vi "Mov_Avg_JS_Dual.vi"(6 "Cycle Length":dbl, 8 "Array In 2":dbl[](array[numeric]), 9 "Input 2":dbl, 10 "Array In":dbl[](array[numeric]), 11 "Input":dbl) -> (0 "Array Out Main 2":dbl[](array[numeric]), 1 "Mean 2":dbl format="%0.2f", 2 "Array Out Main":dbl[](array[numeric]), 3 "Mean":dbl format="%0.2f")   [LabVIEW 2014]
uses:
  <vilib>/Analysis/baseanly.llb/Mean (DBL).vi
  <vilib>/Analysis/NI_AALBase.lvlib
panel:
  # "Moving Average VI"
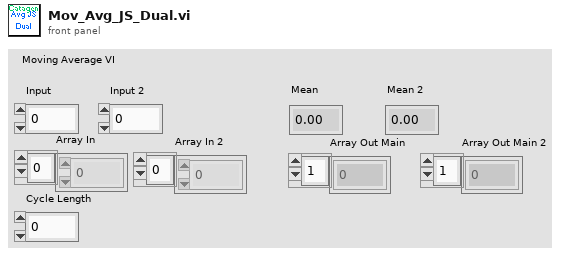
[diagram p1: front panel]
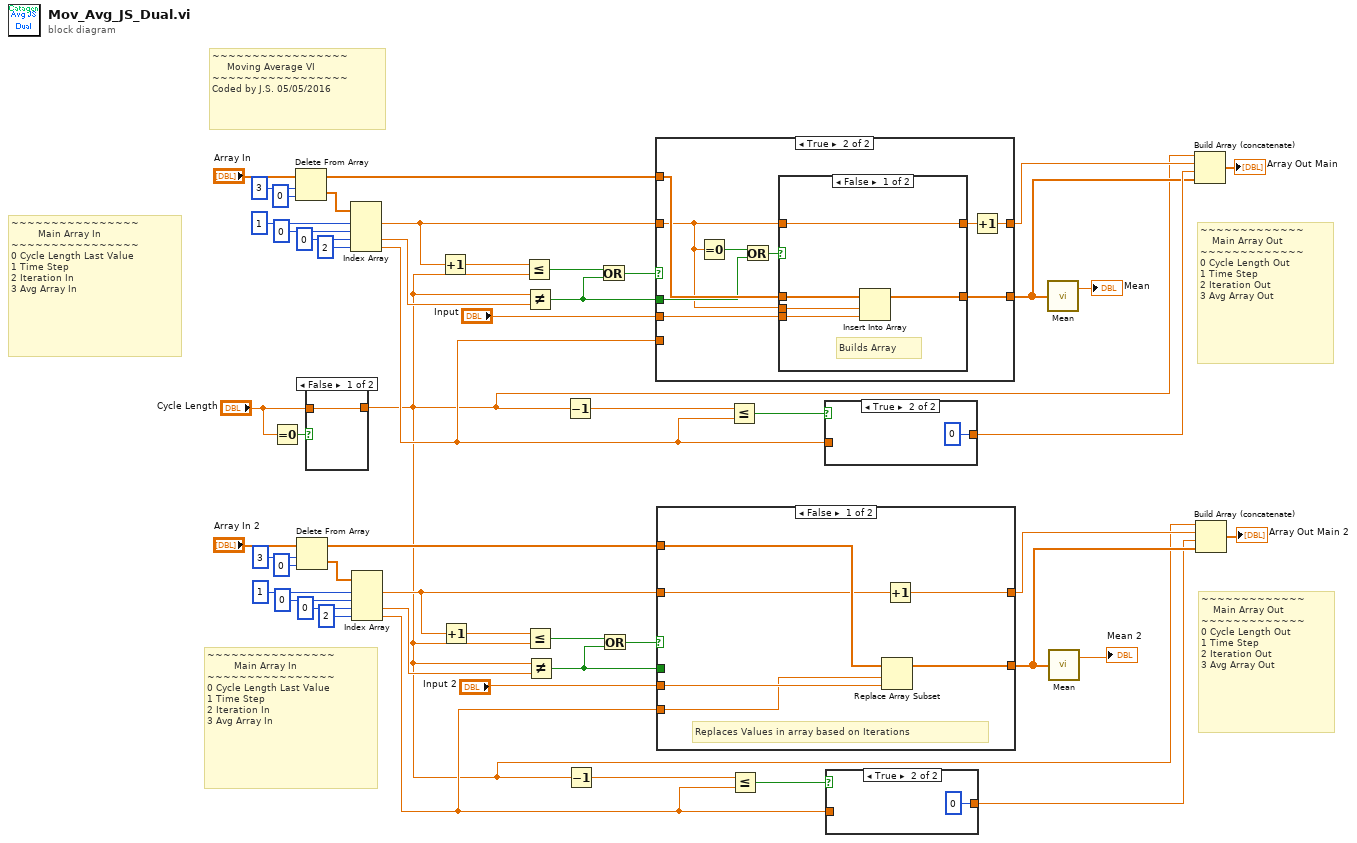
[diagram p0: block diagram]
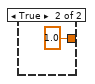
[diagram p2: hidden frame]
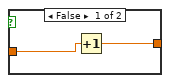
[diagram p3: hidden frame]
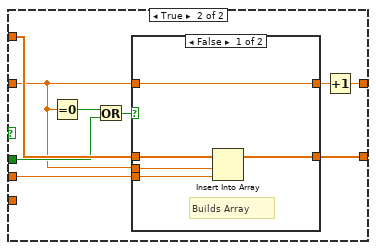
[diagram p4: hidden frame]
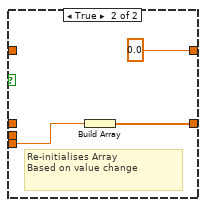
[diagram p5: hidden frame]
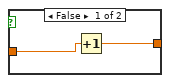
[diagram p6: hidden frame]
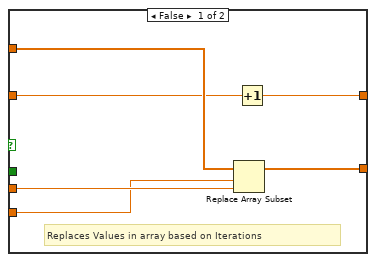
[diagram p7: hidden frame]
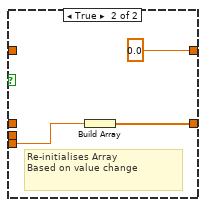
[diagram p8: hidden frame]
diagram:
  # "~~~~~~~~~~~~~~~~\n         Main Array In\n~~~~~~~~~~~~~~~~\n0 Cycle Length Last Value\n1 Time Step\n2 Iteration In\n3 Avg Array In"
  # "~~~~~~~~~~~~~\n    Main Array Out\n~~~~~~~~~~~~~\n0 Cycle Length Out\n1 Time Step\n2 Iteration Out\n3 Avg Array Out"
  # "~~~~~~~~~~~~~~~~\n         Main Array In\n~~~~~~~~~~~~~~~~\n0 Cycle Length Last Value\n1 Time Step\n2 Iteration In\n3 Avg Array In"
  # "~~~~~~~~~~~~~\n    Main Array Out\n~~~~~~~~~~~~~\n0 Cycle Length Out\n1 Time Step\n2 Iteration Out\n3 Avg Array Out"
  # "~~~~~~~~~~~~~~~~~\n     Moving Average VI \n~~~~~~~~~~~~~~~~~\nCoded by J.S. 05/05/2016"
  n1 = Equal To 0?(x="Cycle Length") -> (x = 0?=w3:bool)
  n2 = Delete From Array(array="Array In", length=3, index=0) -> (deleted portion=w41:dbl[], array with subset deleted=w37:dbl[])
  n3 = Delete From Array(array="Array In 2", length=3, index=0) -> (deleted portion=w15:dbl[], array with subset deleted=w18:dbl[])
  n4 = case shown="False" w3 {
    tunnel: "Cycle Length" -> [w52 _]
    tunnel: [w52 1.0 ("Cycle Length")] -> w1
    frame False {
    }
    frame True {
    }
  }
  n5 = Index Array(array=w41, index #1=1 ("index"), index #2=0 ("index"), index #3=0 ("index"), index #4=2 ("index")) -> (element #1=w30:dbl, element #3=w34:dbl, element #4=w32:dbl)  [unwired: 1 out]
  n6 = Index Array(array=w15, index #1=1 ("index"), index #2=0 ("index"), index #3=0 ("index"), index #4=2 ("index")) -> (element #1=w25:dbl, element #3=w21:dbl, element #4=w23:dbl)  [unwired: 1 out]
  n7 = Increment(x=w30) -> (x+1=w29:dbl)
  n8 = Increment(x=w25) -> (x+1=w26:dbl)
  n9 = Less Or Equal?(x=w29, y=w1) -> (x <= y?=w50:bool)
  n10 = Not Equal?(x=w1, y=w34) -> (x != y?=w48:bool)
  n11 = Less Or Equal?(x=w26, y=w1) -> (x <= y?=w9:bool)
  n12 = Not Equal?(x=w1, y=w21) -> (x != y?=w10:bool)
  n13 = Decrement(x=w1) -> (x-1=w46:dbl)
  n14 = Decrement(x=w1) -> (x-1=w12:dbl)
  n15 = Or(x=w50, y=w48) -> (x .or. y?=w51:bool)
  n16 = Or(x=w9, y=w10) -> (x .or. y?=w8:bool)
  n17 = case shown="True" w51 {
    tunnel: "Input" -> [w57 w67]
    tunnel: [w58 w66] -> w43
    tunnel: w37 -> [w59 w68]
    tunnel: w32 -> [w56 _]
    tunnel: w30 -> [w55 w62]
    tunnel: w48 -> [_ w65]
    tunnel: [w54 w61] -> w28
    frame False {
      # "Replaces Values in array based on Iterations"
      n18 = Replace Array Subset(array=w59, new element=w57, index=w56) -> (w58:dbl[])
      n19 = Increment(x=w55) -> (x+1=w54:dbl)
    }
    frame True {
      n20 = Equal To 0?(x=w62) -> (x = 0?=w63:bool)
      n21 = Or(x=w63, y=w65) -> (x .or. y?=w64:bool)
      n22 = case shown="False" w64 {
        tunnel: w68 -> [w73 _]
        tunnel: w67 -> [w72 w75]
        tunnel: [w71 w76] -> w66
        tunnel: w62 -> [w70 _]
        tunnel: w62 -> [w69 _]
        tunnel: [w69 0.0] -> w60
        frame False {
          # "Builds Array"
          n23 = Insert Into Array(array=w73, index=w70, new element=w72) -> (w71:dbl[])
        }
        frame True {
          # "Re-initialises Array\nBased on value change"
          n24 = Build Array(w75) -> (w76:dbl[])
        }
      }
      n25 = Increment(x=w60) -> (x+1=w61:dbl)
    }
  }
  n26 = case shown="False" w8 {
    tunnel: "Input 2" -> [w80 w90]
    tunnel: [w81 w89] -> w14
    tunnel: w18 -> [w82 w91]
    tunnel: w23 -> [w79 _]
    tunnel: w25 -> [w78 w85]
    tunnel: w10 -> [_ w88]
    tunnel: [w77 w84] -> w27
    frame False {
      # "Replaces Values in array based on Iterations"
      n27 = Replace Array Subset(array=w82, new element=w80, index=w79) -> (w81:dbl[])
      n28 = Increment(x=w78) -> (x+1=w77:dbl)
    }
    frame True {
      n29 = Equal To 0?(x=w85) -> (x = 0?=w86:bool)
      n30 = Or(x=w86, y=w88) -> (x .or. y?=w87:bool)
      n31 = case shown="False" w87 {
        tunnel: w91 -> [w96 _]
        tunnel: w90 -> [w95 w98]
        tunnel: [w94 w99] -> w89
        tunnel: w85 -> [w93 _]
        tunnel: w85 -> [w92 _]
        tunnel: [w92 0.0] -> w83
        frame False {
          # "Builds Array"
          n32 = Insert Into Array(array=w96, index=w93, new element=w95) -> (w94:dbl[])
        }
        frame True {
          # "Re-initialises Array\nBased on value change"
          n33 = Build Array(w98) -> (w99:dbl[])
        }
      }
      n34 = Increment(x=w83) -> (x+1=w84:dbl)
    }
  }
  n35 = Less Or Equal?(x=w46, y=w32) -> (x <= y?=w47:bool)
  n36 = Less Or Equal?(x=w12, y=w23) -> (x <= y?=w11:bool)
  n37 = case shown="True" w47 {
    tunnel: [w101 i64 0] -> w44
    tunnel: w32 -> [w100 _]
    frame False {
      n38 = Increment(x=w100) -> (x+1=w101:dbl)
    }
    frame True {
    }
  }
  n39 = case shown="True" w11 {
    tunnel: [w104 i64 0] -> w13
    tunnel: w23 -> [w103 _]
    frame False {
      n40 = Increment(x=w103) -> (x+1=w104:dbl)
    }
    frame True {
    }
  }
  n41 = call-poly <vilib>:"Mean.vi"("X"=w43) -> ("mean"=→"Mean":dbl)  [unwired: 1 out]
  n42 = call-poly <vilib>:"Mean.vi"("X"=w14) -> ("mean"=→"Mean 2":dbl)  [unwired: 1 out]
  n43 = Build Array (concatenate)(w1, w28, w44, w43) -> (→"Array Out Main":dbl[])
  n44 = Build Array (concatenate)(w1, w27, w13, w14) -> (→"Array Out Main 2":dbl[])
